vi "Application_Init.vi"(0 "object in":refnum<class "Application.lvclass">, 5 "error in (no error)":errorcluster) -> (14 "object out":refnum<class "Application.lvclass">, 19 "error out":errorcluster)   [LabVIEW 2019, in "Application.lvclass"]
uses:
  Application.lvclass
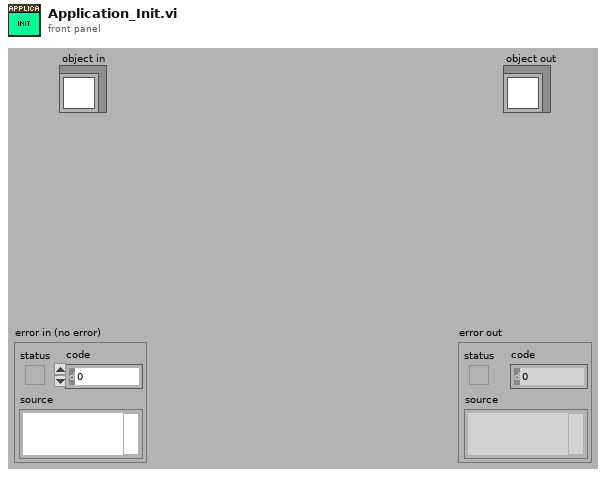
[diagram p1: front panel]
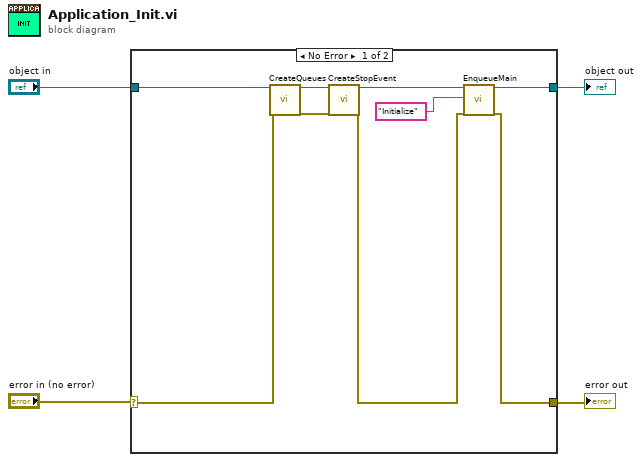
[diagram p0: block diagram]
diagram:
  n1 = case shown="No Error" "error in (no error)" {
    selector: "error in (no error)" -> [w11 w14]
    tunnel: "object in" -> [w10 w15]
    tunnel: [w8 w15] -> w3
    tunnel: [w6 w14] -> w1
    frame No Error {
      n2 = call-dynamic "CreateQueues.vi"("object in"=w10, "error in (no error)"=w11) -> ("object out"=w13:refnum<class "Application.lvclass">, "error out"=w12:errorcluster)  [unwired: 16 in]
      n3 = call "CreateStopEvent.vi"("object in"=w13, "error in (no error)"=w12) -> ("object out"=w9:refnum<class "Application.lvclass">, "error out"=w7:errorcluster)  [unwired: 16 in]
      n4 = call-dynamic "EnqueueMain.vi"("object in"=w9, "Message"="Initialize", "error in (no error)"=w7) -> ("object out"=w8:refnum<class "Application.lvclass">, "error out"=w6:errorcluster)  [unwired: 15 in]
    }
    frame Error {
    }
  }
  "object out" <- w3
  "error out" <- w1
